vi "tacometro.vi"(10 "MÁXIMO \nVALOR":dbl, 11 "VALOR\nACTUAL":dbl) -> (3 "XY Graph":cluster{dbl[], dbl[]}[](graph))   [LabVIEW 2023]
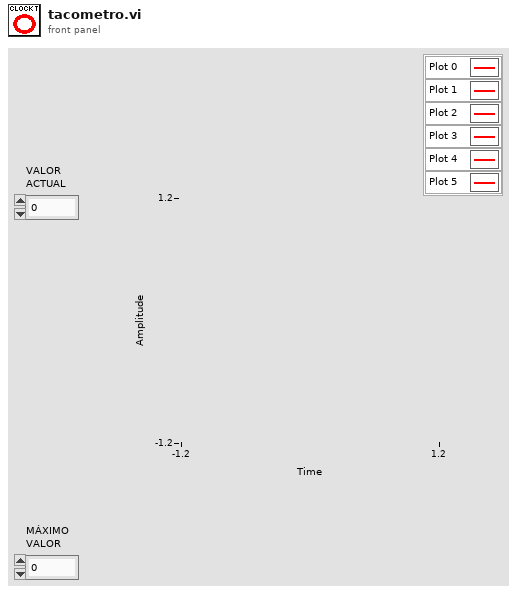
[diagram p1: front panel]
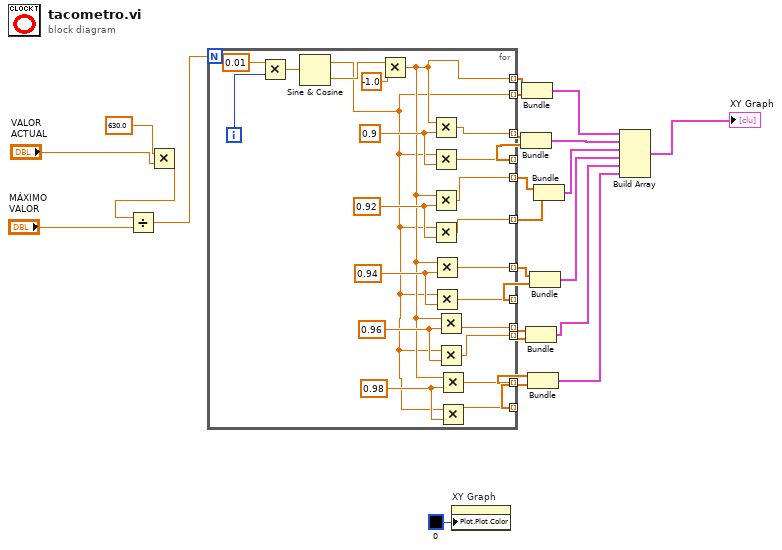
[diagram p0: block diagram]
diagram:
  n1 = Multiply(x=630.0, y="VALOR\nACTUAL") -> (x*y=w23:dbl)
  n2 = Divide(x=w23, y="MÁXIMO \nVALOR") -> (x/y=w25:dbl)
  n3 = for {
    N: w25 -> [_]
    tunnel: [w28] -> w2 mode=indexing
    tunnel: [w29] -> w3 mode=indexing
    tunnel: [w44] -> w7 mode=indexing
    tunnel: [w43] -> w8 mode=indexing
    tunnel: [w39] -> w9 mode=indexing
    tunnel: [w38] -> w10 mode=indexing
    tunnel: [w37] -> w11 mode=indexing
    tunnel: [w36] -> w12 mode=indexing
    tunnel: [w35] -> w13 mode=indexing
    tunnel: [w34] -> w14 mode=indexing
    tunnel: [w27] -> w19 mode=indexing
    tunnel: [w26] -> w20 mode=indexing
    i -> [w31]
    w30 = 0.98 ("y")
    w40 = 0.96 ("y")
    w41 = 0.94 ("y")
    w42 = 0.92 ("y")
    w45 = 0.9 ("y")
    n4 = Multiply(x=0.01 ("y"), y=w31) -> (x*y=w33:dbl)
    n5 = Sine & Cosine(0:w33) -> (1:w28:dbl, 2:w46:dbl)
    n6 = Multiply(x=w46, y=-1.0) -> (x*y=w29:dbl)
    n7 = Multiply(x=w29, y=w45) -> (x*y=w44:dbl)
    n8 = Multiply(x=w28, y=w45) -> (x*y=w43:dbl)
    n9 = Multiply(x=w29, y=w42) -> (x*y=w39:dbl)
    n10 = Multiply(x=w28, y=w42) -> (x*y=w38:dbl)
    n11 = Multiply(x=w29, y=w41) -> (x*y=w37:dbl)
    n12 = Multiply(x=w28, y=w41) -> (x*y=w36:dbl)
    n13 = Multiply(x=w29, y=w40) -> (x*y=w35:dbl)
    n14 = Multiply(x=w28, y=w40) -> (x*y=w34:dbl)
    n15 = Multiply(x=w29, y=w30) -> (x*y=w27:dbl)
    n16 = Multiply(x=w28, y=w30) -> (x*y=w26:dbl)
  }
  n17 = property on="XY Graph" class="XYGraph (strict)"("Plot.Plot Color"=u32 0) -> ()  [unwired: 2 in, 2 out]
  n18 = Bundle(w7, w8) -> (w6:cluster{dbl[], dbl[]})  [unwired: 1 in]
  n19 = Bundle(w3, w2) -> (w5:cluster{dbl[], dbl[]})  [unwired: 1 in]
  n20 = Bundle(w13, w14) -> (w17:cluster{dbl[], dbl[]})  [unwired: 1 in]
  n21 = Bundle(w19, w20) -> (w18:cluster{dbl[], dbl[]})  [unwired: 1 in]
  n22 = Bundle(w11, w12) -> (w16:cluster{dbl[], dbl[]})  [unwired: 1 in]
  n23 = Bundle(w9, w10) -> (w15:cluster{dbl[], dbl[]})  [unwired: 1 in]
  n24 = Build Array(w5, w6, w15, w16, w17, w18) -> (→"XY Graph":cluster{dbl[], dbl[]}[])
